vi "Test Case, Is IPG Shutdown.vi"() -> ()   [LabVIEW 2010]
uses:
  Charger/Charger_Status Control.ctl
  Drivers/Charger Test Set/Charger_Input Control.ctl
panel:
  in  "idle":bool
  out "Charge Status":T1={"MICS ID"=4417, "VBAT"=nan, "ChargingState"="", "VBAT Slide"=3.5, "Status"="", "TemperatureLevel"=nan, "IPG_ReceivedLevel"=nan, "VBAT Target"=nan, "Charger Setpoint"=nan, "Index"=0, "Ready"=TRUE, "Charger Inputs"={"address"="COM17", "position"=0, "setpoint"=7500.0}, "MICS Inputs"={"address"="", "chan"=2, "ID"=0}} {"MICS Inputs"."ID" format="%04x"; "MICS Inputs"."chan" min=1 max=10 step=1; "Charger Inputs"."setpoint" min=0.0 max=20000.0 step=100.0; "Charger Inputs"."position" min=0 max=5 step=1; "MICS ID" format="%04x"; "VBAT Target" format="%.2f"; "VBAT Slide" scale=3.5..4.0 scale format="%.2f"; "VBAT" format="%.2f"}
  out "error out":errorcluster
  in  "error in":errorcluster
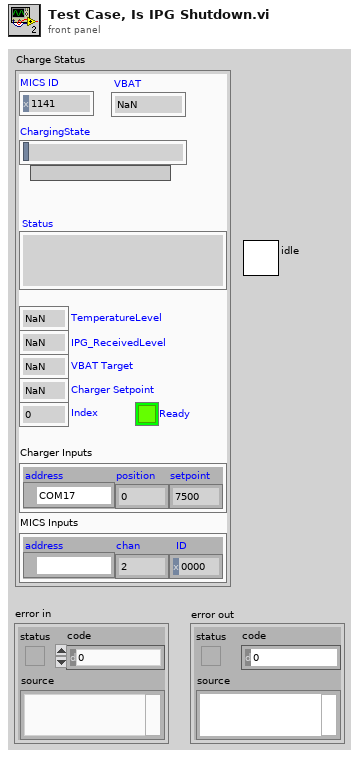
[diagram p1: front panel]
types:
  T1 = typedef "Charger_Status Control.ctl" = cluster{"MICS ID":u32, "VBAT":dbl, "ChargingState":string, "VBAT Slide":dbl, "Status":string, "TemperatureLevel":dbl, "IPG_ReceivedLevel":dbl, "VBAT Target":dbl, "Charger Setpoint":dbl, "Index":i32, "Ready":bool, "Charger Inputs":T2, "MICS Inputs":cluster{"address":refnum<visa-resource-name>, "chan":u16, "ID":u32}}
  T2 = typedef "Charger_Input Control.ctl" = cluster{"address":refnum<visa-resource-name>, "position":i32, "setpoint":dbl}
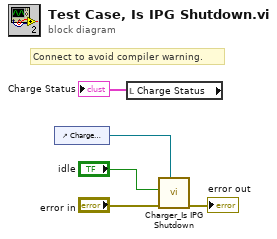
[diagram p0: block diagram]
diagram:
  # "Connect to avoid compiler warning."
  n1 = control-ref of="Charge Status"() -> (w2:refnum<vi>)
  n2 = local read "Charge Status"() -> (→"Charge Status":T1)
  n3 = call "Charger_Is IPG Shutdown.vi"("Status Refnum"=w2, "error in"="error in", "idle"="idle") -> ("error out"=→"error out":errorcluster)  [unwired: 6 in]
